vi "Test API.vi"   [LabVIEW 2018]
uses:
  src/api/logger_class/Log Levels.ctl
  6cc74522-22c2-4448-8e2a-3359a5076545.vi
  9b32b05d-753e-4f65-8e2e-4f66a2a2a8f6.vi
  d2d7bf56-c2ec-45ee-8ddd-ee23ec9d339c.vi
  3e1e885e-64a1-4c1c-bc84-8c9983270b1a.vi
  64102c65-737f-4366-b704-a46cb2200817.vi
  9bdd3682-e6cc-44bd-88aa-3770d79584fc.vi
  6caa08eb-ef88-4ec6-8e27-2b667660373f.vi
  704a625a-bf60-40cc-a4c4-2e9e31a30157.vi
  9a2171c2-14ed-41aa-a883-74703c5961df.vi
  a6761f4a-cf0a-4387-b992-fcbb2724d4f1.vi
  63695a67-f777-48d7-8ca3-c506280cf678.vi
  c8782fa7-858e-4347-a21d-ce57f127006c.vi
  0ca037f3-c2eb-4335-b5e9-525bdf736c9a.vi
  3f533fa5-397a-4888-a51d-ab0877a39b27.vi
  06261af6-0207-4d6a-a0b5-68d7330c5dc2.vi
  29a6184c-9645-462b-b41d-e9b5e971689b.vi
  f437223c-2033-4ec3-ba5c-fdf367536402.vi
  51edc14d-fb83-4451-bde2-8a786fcee62f.vi
  6cc74522-22c2-4448-8e2a-3359a5076545.vi/bae24b8d-f663-491e-8374-2218e527d0d0.vi
  9b32b05d-753e-4f65-8e2e-4f66a2a2a8f6.vi/d00d689c-c4e8-4614-912e-44cd26a3e5a1.vi
  d2d7bf56-c2ec-45ee-8ddd-ee23ec9d339c.vi/aa8de69b-4483-4f14-98ed-40fb95e7c15f.vi
  3e1e885e-64a1-4c1c-bc84-8c9983270b1a.vi/0f5afe7c-e05d-4549-afb0-2c08b5afa0c9.vi
  64102c65-737f-4366-b704-a46cb2200817.vi/35b039e2-05a6-4d5d-95fc-f9607323732b.vi
  9bdd3682-e6cc-44bd-88aa-3770d79584fc.vi/1f4baa75-7c2a-40e9-b4bc-d287912a8f57.vi
  6caa08eb-ef88-4ec6-8e27-2b667660373f.vi/bae24b8d-f663-491e-8374-2218e527d0d0.vi
  704a625a-bf60-40cc-a4c4-2e9e31a30157.vi/a02c6254-97f5-44e3-a3a9-7fdb6dfbd055.vi
  9a2171c2-14ed-41aa-a883-74703c5961df.vi/caf2d4a3-5a7b-40e1-b7b0-74b52901b9f9.vi
  a6761f4a-cf0a-4387-b992-fcbb2724d4f1.vi/a06e9705-c341-4fd3-ab56-b0df9b5f3d25.vi
  63695a67-f777-48d7-8ca3-c506280cf678.vi/5a01e313-fc7d-4519-ba39-81d8e4580f6b.vi
  c8782fa7-858e-4347-a21d-ce57f127006c.vi/5ce1af88-85f0-419a-8d80-1694d27860f0.vi
  29a6184c-9645-462b-b41d-e9b5e971689b.vi/0a1ee2ab-da6d-4243-8cf3-8125e611a602.vi
  f437223c-2033-4ec3-ba5c-fdf367536402.vi/73f0ec31-6bdf-4568-9d3b-fef50ac01b30.vi
  51edc14d-fb83-4451-bde2-8a786fcee62f.vi/6f202c45-f0ca-42f4-9f63-a87d9fe0c32d.vi
  6cc74522-22c2-4448-8e2a-3359a5076545.vi/bae24b8d-f663-491e-8374-2218e527d0d0.vi/6f202c45-f0ca-42f4-9f63-a87d9fe0c32d.vi
  9b32b05d-753e-4f65-8e2e-4f66a2a2a8f6.vi/d00d689c-c4e8-4614-912e-44cd26a3e5a1.vi/73f0ec31-6bdf-4568-9d3b-fef50ac01b30.vi
  d2d7bf56-c2ec-45ee-8ddd-ee23ec9d339c.vi/aa8de69b-4483-4f14-98ed-40fb95e7c15f.vi/0a1ee2ab-da6d-4243-8cf3-8125e611a602.vi
  6caa08eb-ef88-4ec6-8e27-2b667660373f.vi/bae24b8d-f663-491e-8374-2218e527d0d0.vi/6f202c45-f0ca-42f4-9f63-a87d9fe0c32d.vi
  704a625a-bf60-40cc-a4c4-2e9e31a30157.vi/a02c6254-97f5-44e3-a3a9-7fdb6dfbd055.vi/73f0ec31-6bdf-4568-9d3b-fef50ac01b30.vi
  9a2171c2-14ed-41aa-a883-74703c5961df.vi/caf2d4a3-5a7b-40e1-b7b0-74b52901b9f9.vi/0a1ee2ab-da6d-4243-8cf3-8125e611a602.vi
  src/api/configuration/filters/data_item_filter/Data Item.lvclass
  C:/Users/Colin/Documents/software_projects/labview/glog/src/api/extension/filter_interface/Filter.lvclass
  src/api/configuration/filters/regex_filter/Regex.lvclass
  src/registry/Enable All.vi
  src/registry/Disable All.vi
  src/api/configuration/filters/data_item_filter/New (Element).vi
  src/api/configuration/filters/regex_filter/New (Element).vi
  src/api/configuration/scopes/basic_scope/New (Element).vi
  src/api/logger_class/Log (Log Record).vi
  src/api/logger_class/Log (Parts).vi
  <vilib>/ErrorRing/Error Ring.xnode
  src/api/GLog.lvlib
  src/api/configuration/filters/combination_filter/Combination.lvclass
  src/api/logger_class/Logger.lvclass
  src/api/configuration/scopes/basic_scope/Basic.lvclass
  src/api/configuration/handlers/file_handler/File Handler.lvclass
  src/api/configuration/handlers/string_handler/String Handler.lvclass
  src/api/configuration/formatters/JSON_formatter/JSON.lvclass
  src/api/configuration/formatters/format_string_formatter/Format String.lvclass
types:
  T1 = typedef "GLog.lvlib/Logger.lvclass/Log Levels.ctl" = enum16{"Trace", "Debug", "Info", "Warning", "Error", "Critical"}
  T2 = typedef "GLog.lvlib/Logger.lvclass/Log Record.ctl" = cluster{"level":T3, "timestamp":timestamp, "call chain":string[], "message":string, "data":variant}
  T3 = typedef "GLog.lvlib/Logger.lvclass/Internal Log Levels.ctl" = enum16{"Trace", "Debug", "Info", "Warning", "Error", "Critical", "Internal"}
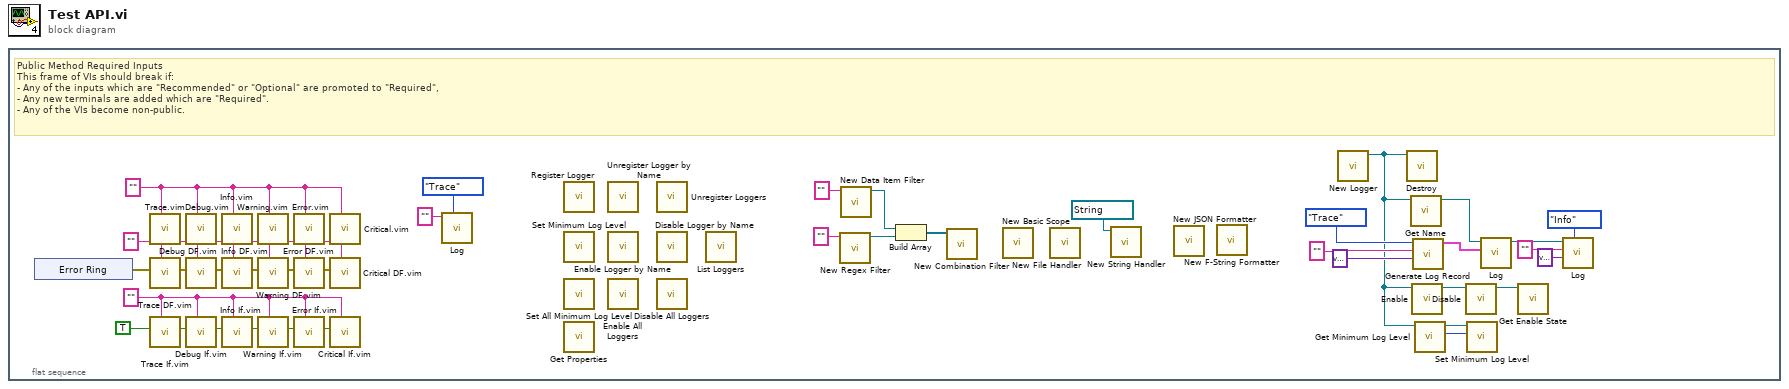
[diagram p0: block diagram]
diagram:
  n1 = flat-sequence {
    frame #0 {
      w35 = "" ("message")
      w36 = "" ("message")
      w37 = "" ("message")
      # "Public Method Required Inputs\nThis frame of VIs should break if:\n- Any of the inputs which are \"Recommended\" or \"Optional\" are promoted to \"Required\", \n- Any new terminals are added which are \"Required\".\n- Any of the VIs become non-public."
      n2 = xnode "Error Ring"() -> ("error out"=w18:errorcluster)
      n3 = call "Trace.vim"("message"=w37) -> ()  [unwired: 10 in, 1 out]
      n4 = call "Trace DF.vim"("message"=w36, "dataflow in"=w18) -> ("dataflow out"=w28:errorcluster)  [unwired: 9 in]
      n5 = call "Trace If.vim"("message"=w35, "condition in"=TRUE) -> ("condition out"=w33:bool)  [unwired: 9 in]
      n6 = call "Debug.vim"("message"=w37) -> ()  [unwired: 10 in, 1 out]
      n7 = call "Debug DF.vim"("message"=w36, "dataflow in"=w28) -> ("dataflow out"=w27:errorcluster)  [unwired: 9 in]
      n8 = call "Debug If.vim"("message"=w35, "condition in"=w33) -> ("condition out"=w32:bool)  [unwired: 9 in]
      n9 = call "Info.vim"("message"=w37) -> ()  [unwired: 10 in, 1 out]
      n10 = call "Info DF.vim"("message"=w36, "dataflow in"=w27) -> ("dataflow out"=w26:errorcluster)  [unwired: 9 in]
      n11 = call "Info If.vim"("message"=w35, "condition in"=w32) -> ("condition out"=w31:bool)  [unwired: 9 in]
      n12 = call "Warning.vim"("message"=w37) -> ()  [unwired: 10 in, 1 out]
      n13 = call "Warning DF.vim"("message"=w36, "dataflow in"=w26) -> ("dataflow out"=w25:errorcluster)  [unwired: 9 in]
      n14 = call "Warning If.vim"("message"=w35, "condition in"=w31) -> ("condition out"=w30:bool)  [unwired: 9 in]
      n15 = call "Error.vim"("message"=w37) -> ()  [unwired: 10 in, 1 out]
      n16 = call "Error DF.vim"("message"=w36, "dataflow in"=w25) -> ("dataflow out"=w24:errorcluster)  [unwired: 9 in]
      n17 = call "Error If.vim"("message"=w35, "condition in"=w30) -> ("condition out"=w29:bool)  [unwired: 9 in]
      n18 = call "Critical.vim"("message"=w37) -> ()  [unwired: 10 in, 1 out]
      n19 = call "Critical DF.vim"("message"=w36, "dataflow in"=w24) -> ()  [unwired: 9 in, 1 out]
      n20 = call "Critical If.vim"("message"=w35, "condition in"=w29) -> ()  [unwired: 9 in, 1 out]
      n21 = call "Log.vi"("severity"=Log_Levels."Trace", "message"="") -> ()  [unwired: 10 in]
      n22 = call "Register Logger.vi"() -> ()  [unwired: 11 in, 1 out]
      n23 = call "Set Minimum Log Level.vi"() -> ()  [unwired: 11 in, 1 out]
      n24 = call "Set All Minimum Log Level.vi"() -> ()  [unwired: 11 in, 1 out]
      n25 = call "Get Properties.vi"() -> ()  [unwired: 10 in, 2 out]
      n26 = call "Unregister Logger by Name.vi"() -> ()  [unwired: 10 in, 2 out]
      n27 = call "Enable Logger by Name.vi"() -> ()  [unwired: 11 in, 1 out]
      n28 = call "Enable All Loggers.vi"() -> ()  [unwired: 11 in, 1 out]
      n29 = call "Unregister Loggers.vi"() -> ()  [unwired: 10 in, 2 out]
      n30 = call "Disable Logger by Name.vi"() -> ()  [unwired: 11 in, 1 out]
      n31 = call "Disable All Loggers.vi"() -> ()  [unwired: 11 in, 1 out]
      n32 = call "List Loggers.vi"() -> ()  [unwired: 10 in, 2 out]
      n33 = call-poly "New Regex Filter.vi"("regex string"="") -> ("regex out"=w20:refnum<class "Regex.lvclass">)  [unwired: 9 in, 1 out]
      n34 = call-poly "New Data Item Filter.vi"("data item name"="") -> ("data item out"=w21:refnum<class "Data Item.lvclass">)  [unwired: 9 in, 1 out]
      n35 = Build Array(w21, w20) -> (w19:refnum<class "Filter.lvclass">[])
      n36 = call "New Combination Filter.vi"("sub-filters"=w19) -> ()  [unwired: 10 in, 1 out]
      n37 = call-poly "New Basic Scope.vi"() -> ()  [unwired: 11 in, 1 out]
      n38 = call "New File Handler.vi"() -> ()  [unwired: 11 in, 1 out]
      n39 = call "New String Handler.vi"("string control"=refnum<vi> refnum) -> ()  [unwired: 10 in, 1 out]
      n40 = call "New JSON Formatter.vi"() -> ()  [unwired: 11 in, 1 out]
      n41 = call "New F-String Formatter.vi"() -> ()  [unwired: 11 in, 1 out]
      n42 = call "New Logger.vi"() -> ("logger"=w3:refnum<class "Logger.lvclass">)  [unwired: 10 in, 1 out]
      n43 = call "Destroy.vi"("logger in"=w3) -> ()  [unwired: 9 in, 2 out]
      n44 = call "Get Name.vi"("logger in"=w3) -> ("logger out"=w8:refnum<class "Logger.lvclass">)  [unwired: 9 in, 1 out]
      n45 = call "Enable.vi"("logger in"=w3) -> ("logger out"=w5:refnum<class "Logger.lvclass">)  [unwired: 10 in]
      n46 = call "Generate Log Record.vi"("data"=variant, "message"="", "log level"=Log_Levels."Trace") -> ("log record"=w9:T2)  [unwired: 8 in]
      n47 = call "Get Minimum Log Level.vi"("logger in"=w3) -> ("minimum log level"=w2:T1, "logger out"=w1:refnum<class "Logger.lvclass">)  [unwired: 9 in]
      n48 = call "Disable.vi"("logger in"=w5) -> ("logger out"=w4:refnum<class "Logger.lvclass">)  [unwired: 10 in]
      n49 = call "Set Minimum Log Level.vi"("minimum log level"=w2, "logger in"=w1) -> ()  [unwired: 9 in, 1 out]
      n50 = call-poly "Log.vi"("log record"=w9, "logger in"=w8) -> ("logger out"=w7:refnum<class "Logger.lvclass">)  [unwired: 9 in]
      n51 = call "Get Enable State.vi"("logger in"=w4) -> ()  [unwired: 9 in, 2 out]
      n52 = call-poly "Log.vi"("log level"=Log_Levels."Info", "data (null)"=variant, "message"="", "logger in"=w7) -> ()  [unwired: 7 in, 1 out]
    }
  }
